vi "Split Tasks.vi"(0 "Task Specification Array":T2[](array[typedef]) {"Channels"."Terminal configuration" items=["Default"=-1, "RSE"=10083, "Differential"=10106, "Pseudodifferential"=12529]}) -> (3 "Sync Task":T1, 4 "AO Tasks":T1[](array[typedef]), 14 "DI Tasks":T1[](array[typedef]), 15 "AI Tasks":T1[](array[typedef]))   [LabVIEW 2020]
uses:
  Type Defs/Task Struct.ctl
  Type Defs/Task Specification Struct.ctl
  Type Defs/Channel Struct.ctl
panel:
  in  "Dummy task":T1
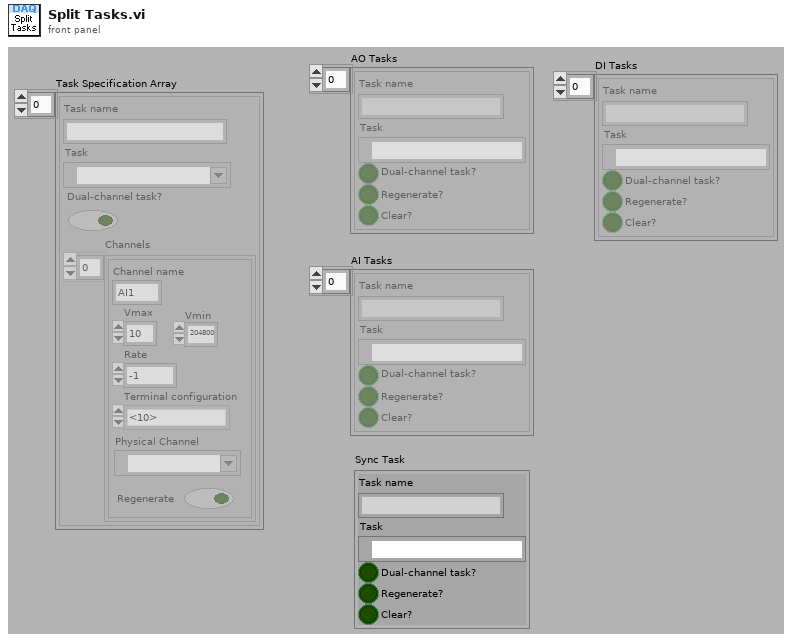
[diagram p1: front panel]
types:
  T1 = typedef "Task Struct.ctl" = cluster{"Task name":string, "Task":refnum<k21>, "Dual-channel task?":bool, "Regenerate?":bool, "Clear?":bool}
  T2 = typedef "Task Specification Struct.ctl" = cluster{"Task name":string, "Task":refnum<k21>, "Dual-channel task?":bool, "Channels":T3[]}
  T3 = typedef "Channel Struct.ctl" = cluster{"Channel name":string, "Vmax":dbl, "Vmin":dbl, "Rate":dbl, "Terminal configuration":i32, "Physical Channel":tag, "Regenerate":bool}
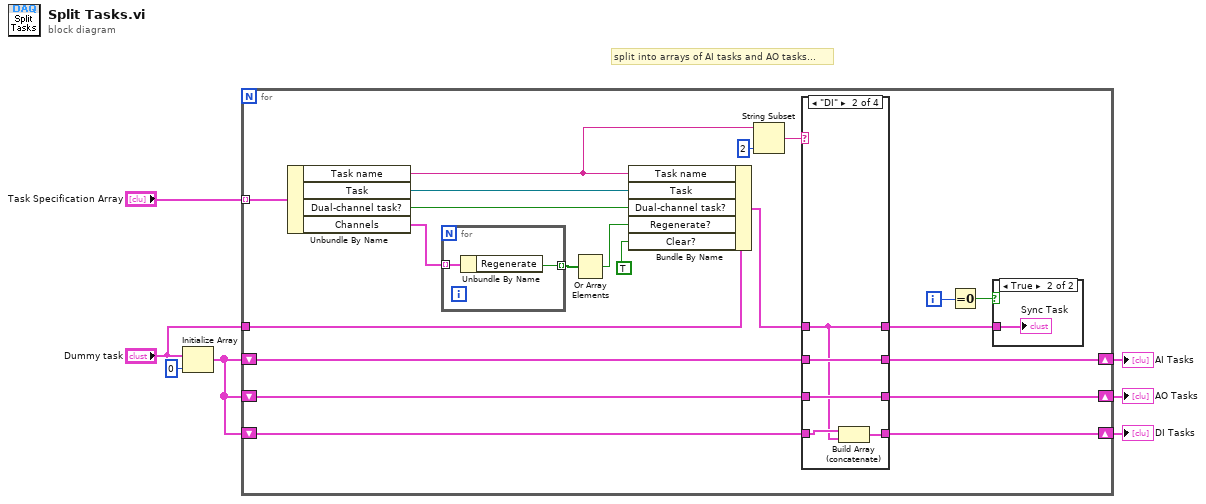
[diagram p0: block diagram]
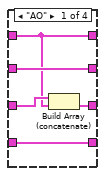
[diagram p3: hidden frame]
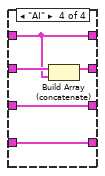
[diagram p5: hidden frame]
diagram:
  # "split into arrays of AI tasks and AO tasks..."
  n1 = Initialize Array("Dummy task", 0 ("dimension size")) -> (w2:T1[])
  n2 = for {
    tunnel: "Task Specification Array" -> [w28] mode=indexing
    shift-right: [w24] -> w4
    shift-left: w2 -> [w25]
    shift-right: [w22] -> w5
    shift-left: w2 -> [w23]
    tunnel: "Dummy task" -> [w17]
    shift-right: [w8] -> w1
    shift-left: w2 -> [w9]
    i -> [w15]
    n3 = Unbundle By Name(w28) -> ("Task name"=w20:string, "Task"=w19:refnum<k21>, "Dual-channel task?"=w18:bool, "Channels"=w13:T3[])
    n4 = for {
      tunnel: w13 -> [w30] mode=indexing
      tunnel: [w29] -> w12 mode=indexing
      n5 = Unbundle By Name(w30) -> ("Regenerate"=w29:bool)
    }
    n6 = Or Array Elements(Boolean array=w12) -> (logical OR=w11:bool)
    n7 = Bundle By Name(cluster=w17, "Task name"=w20, "Task"=w19, "Dual-channel task?"=w18, "Regenerate?"=w11, "Clear?"=TRUE) -> (w16:T1)
    n8 = String Subset(string=w20, length (rest)=2 ("length (rest)")) -> (substring=w26:string)  [unwired: 1 in]
    n9 = case shown="\"DI\"" w26 {
      tunnel: w25 -> [w34 w41 w45 w49]
      tunnel: [w34 w41 w45 w48] -> w24
      tunnel: w23 -> [w36 w40 w44 w50]
      tunnel: [w35 w40 w44 w50] -> w22
      tunnel: [w33 w37 w43 w47] -> w21
      tunnel: w16 -> [w33 w37 w43 w47]
      tunnel: w9 -> [w32 w39 w42 w46]
      tunnel: [w32 w38 w42 w46] -> w8
      frame "AO" {
        n10 = Build Array (concatenate)(w36, w33) -> (w35:T1[])
      }
      frame "DI" {
        n11 = Build Array (concatenate)(w39, w37) -> (w38:T1[])
      }
      frame Default {
      }
      frame "AI" {
        n12 = Build Array (concatenate)(w49, w47) -> (w48:T1[])
      }
    }
    n13 = Equal To 0?(x=w15) -> (x = 0?=w14:bool)
    n14 = case shown="True" w14 {
      tunnel: w21 -> [_ w31]
      frame False {
      }
      frame True {
        "Sync Task" <- w31
      }
    }
  }
  "AO Tasks" <- w5
  "AI Tasks" <- w4
  "DI Tasks" <- w1
